vi "Get wavefrom subset absolute time.vi"(8 "error in (no error)":errorcluster, 9 "Waveform":waveform(dbl), 10 "Duration [s]":dbl, 11 "Start Time [s]":dbl) -> (0 "error out":errorcluster, 1 "Waveform subset":waveform(dbl))   [LabVIEW 2013]
uses:
  <vilib>/Waveform/WDTOps.llb/WDT Get Waveform Subset DBL.vi
panel:
  out "dt":dbl
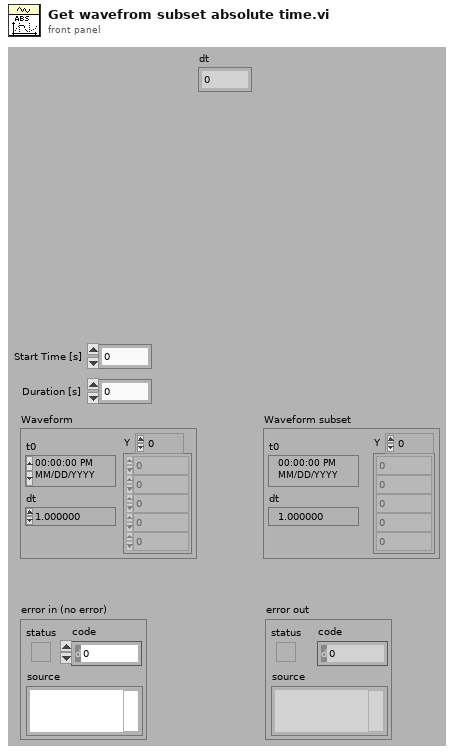
[diagram p1: front panel]
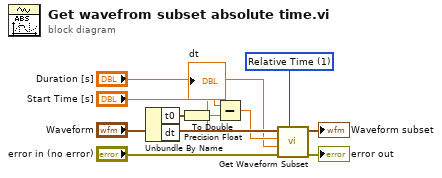
[diagram p0: block diagram]
diagram:
  w5 = u16 1 items=["Samples", "Relative Time"] ("start/duration format")
  n1 = Unbundle By Name("Waveform") -> ("t0"=w7:timestamp, "dt"=→"dt":dbl)
  n2 = To Double Precision Float(number=w7) -> (double precision float=w8:dbl)
  n3 = Subtract(x="Start Time [s]", y=w8) -> (x-y=w9:dbl)
  n4 = call-poly <vilib>:"Get Waveform Subset.vi"("start/duration format"=w5, "error in (no error)"="error in (no error)", "duration"="Duration [s]", "start samples/time"=w9, "waveform in"="Waveform") -> ("error out"=→"error out":errorcluster, "waveform out"=→"Waveform subset":waveform(dbl))  [unwired: 1 in, 2 out]
